vi "FileList.vi"(0 "VISA Refnum in":refnum<visa-resource-name>="COM1", 5 "delay File List":u32=500, 7 "string to write":string="*IDN?\n") -> (15 "Array":string[](array[string]))   [LabVIEW 2012]
uses:
  <vilib>/Instr/_visa.llb/VISA Configure Serial Port (Instr).vi
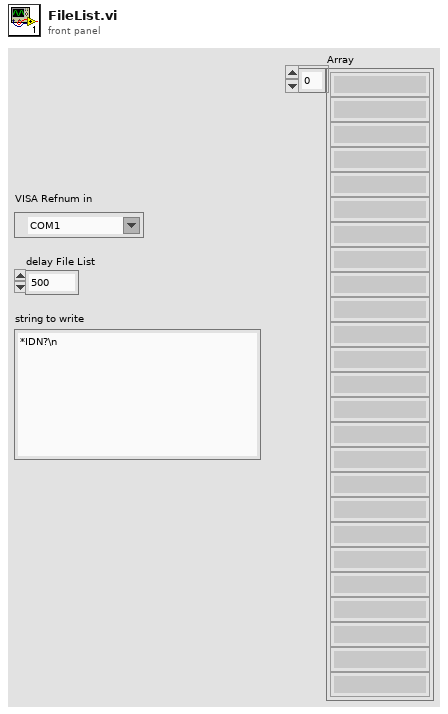
[diagram p1: front panel]
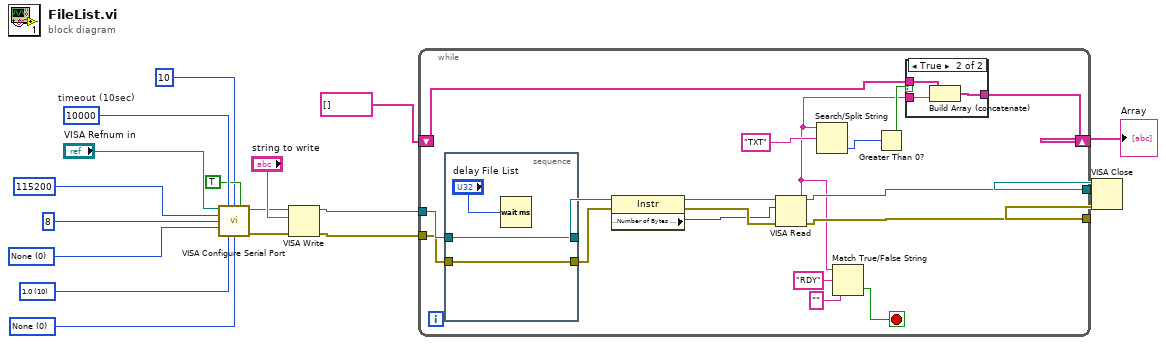
[diagram p0: block diagram]
diagram:
  w18 = u16 0 items=["None"=0, "XON/XOFF"=1, "RTS/CTS"=2, "DTR/DSR"=4] ("flow control")
  w17 = u16 10 items=["1.0"=10, "1.5"=15, "2.0"=20] ("stop bits")
  w16 = u16 0 items=["None", "Odd", "Even", "Mark", "Space"] ("parity")
  w12 = u32 10000  # timeout (10sec)
  n1 = call-poly "VISA Configure Serial Port"("VISA resource name"="VISA Refnum in", "timeout (10sec)"=w12, "termination char\n(0xA = '\\n' = LF)"=u8 10 ("termination char\n(0xA = '\\n' = LF)"), "Enable Termination\nChar (T)"=TRUE ("Enable Termination\nChar (T)"), "baud rate (9600)"=u32 115200 ("baud rate"), "data bits (8)"=u16 8 ("data bits"), "parity (0:none)"=w16, "stop bits (10: 1 bit)"=w17, "flow control (0:none)"=w18) -> ("VISA resource name out"=w10:refnum<visa-resource-name>, "error out"=w9:errorcluster)  [unwired: 1 in, 4 out]
  n2 = VISA Write(VISA resource name=w10, write buffer="string to write", error in (no error)=w9) -> (VISA resource name out=w4:refnum<visa-resource-name>, error out=w3:errorcluster)  [unwired: 1 out]
  n3 = while {
    tunnel: [w33] -> w6
    tunnel: [w32] -> w5
    tunnel: w4 -> [w26]
    tunnel: w3 -> [w25]
    shift-right: [w23] -> w1
    shift-left: string[] [] -> [w24]
    stop <- w30 stop-if-true
    n4 = stacked-sequence {
      tunnel: w25 -> [w43]
      tunnel: [w43] -> w27
      tunnel: w26 -> [w42]
      tunnel: [w42] -> w28
      frame #0 {
        n5 = Wait (ms)(milliseconds to wait="delay File List") -> ()  [unwired: 1 out]
      }
    }
    n6 = property class="Instr"(reference=w28, error in=w27) -> (reference out=w36:refnum<visa-resource-name>, error out=w35:errorcluster, "Serial Settings:Number of Bytes at Serial Port"=w34:u32)
    n7 = VISA Read(VISA resource name=w36, byte count=w34, error in (no error)=w35) -> (VISA resource name out=w33:refnum<visa-resource-name>, read buffer=w19:string, error out=w32:errorcluster)  [unwired: 1 out]
    n8 = Search/Split String(string=w19, search string/char (-)="TXT") -> (offset of match=w21:i32)  [unwired: 1 in, 2 out]
    n9 = Match True/False String(2:"" ("false string"), 3:"RDY" ("true string"), 4:w19) -> (0:w30:bool)  [unwired: 1 out]
    n10 = Greater Than 0?(x=w21) -> (x > 0?=w20:bool)
    n11 = case shown="True" w20 {
      tunnel: w24 -> [w37 w40]
      tunnel: [w37 w39] -> w23
      tunnel: w19 -> [_ w38]
      frame False {
      }
      frame True {
        n12 = Build Array (concatenate)(w40, w38) -> (w39:string[])
      }
    }
  }
  "Array" <- w1
  n13 = VISA Close(VISA resource name=w6, error in (no error)=w5) -> ()  [unwired: 1 out]
